vi "Bayer12bit.vi"() -> ()   [LabVIEW 2022 SP3]
uses:
  <vilib>/vision/NI_Vision_Development_Module.lvlib
panel:
  out "Binary Threshold":T1(plugin-control)
  in  "Range":cluster{"Lower value":sgl, "Upper value":sgl}={"Lower value"=128.0, "Upper value"=255.0} {"Upper value" format="%.2f"; "Lower value" format="%.2f"}
  in  "Color Plane":i32(ring)=1 items=["Red", "Green", "Blue", "Hue", "Saturation", "Luminance", "Value", "Intensity"]
  out "Color Plane Extract":T1(plugin-control)
  in  "Bit Depth (0)":u32=12
  out "Processing Time":u32
  in  "RUN":bool
  out "RGB":T1(plugin-control)
  in  "Bayer Parameters":T2={"Pattern"=3, "Algorithm"=0, "Red Gain"=1.0, "Green Gain"=1.0, "Blue Gain"=1.0} {"Blue Gain" format="%_4g"; "Green Gain" format="%_4g"; "Red Gain" format="%_4g"; "Algorithm" items=["Bilinear", "VNG"]; "Pattern" items=["GB", "GR", "BG", "RG"]}
  in  "Stop":bool
  out "Original":T1(plugin-control)
  in  "File Path":path=path "C:/Users/au540322/Documents/Projects/BioDiscover/src/LabVIEW/resources/BayerImages/OriginalBayer.png"
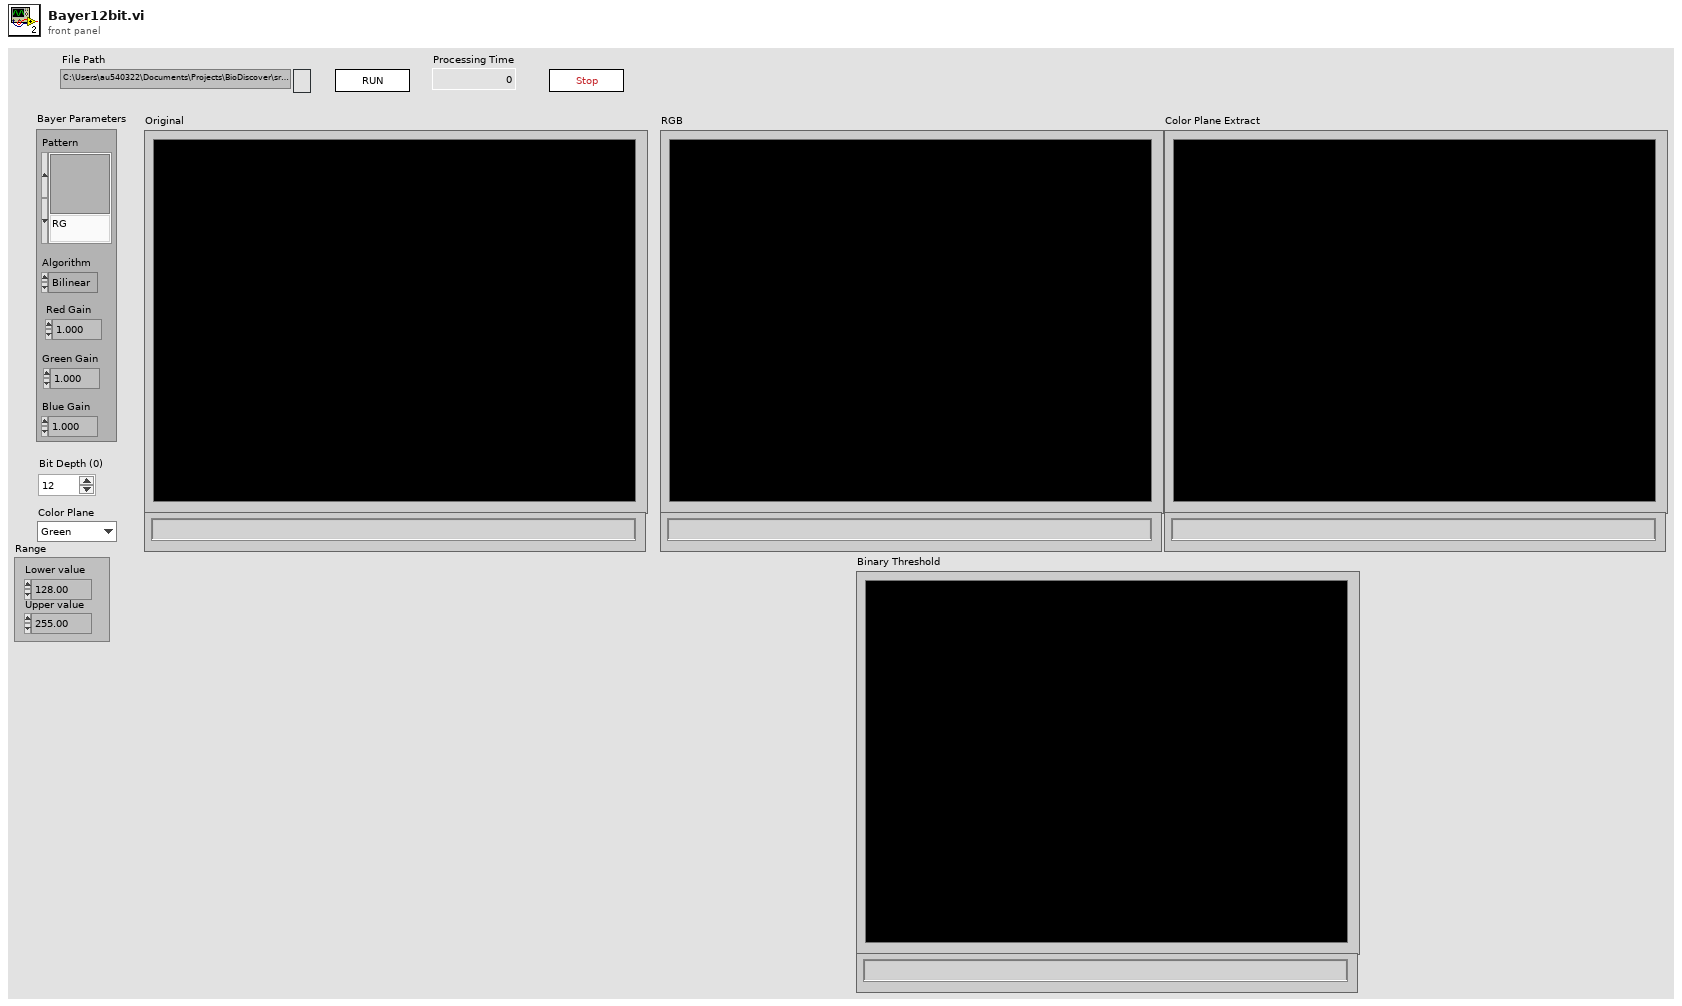
[diagram p1: front panel]
types:
  T1 = typedef "IMAQ Image.ctl" = refnum<image>
  T2 = cluster{"Pattern":i32, "Algorithm":i32, "Red Gain":dbl, "Green Gain":dbl, "Blue Gain":dbl}
  T3 = typedef "Image Type" = u32
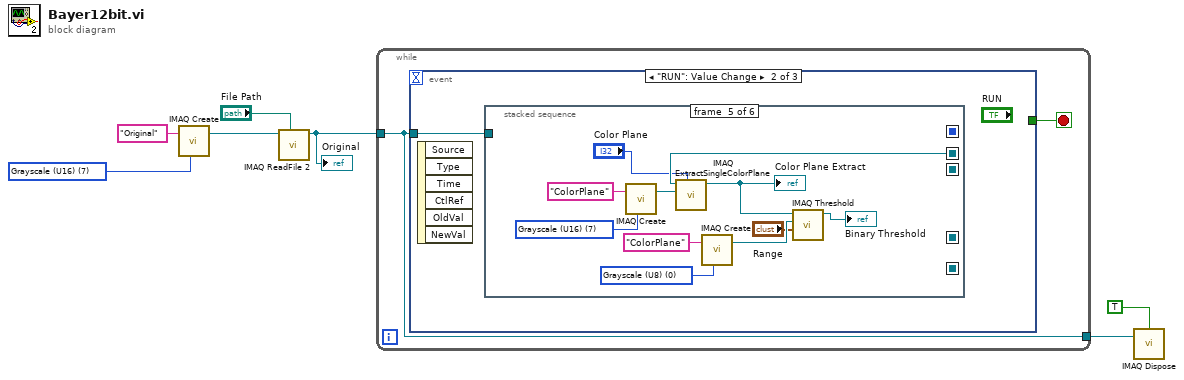
[diagram p0: block diagram]
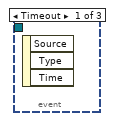
[diagram p2: hidden frame]
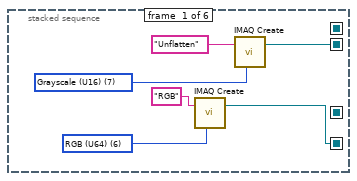
[diagram p3: hidden frame]
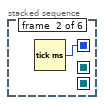
[diagram p4: hidden frame]
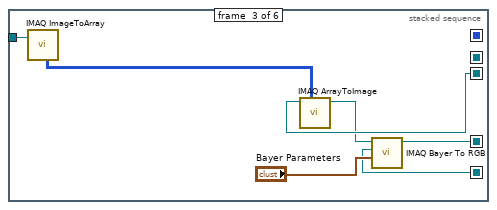
[diagram p5: hidden frame]
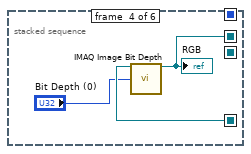
[diagram p6: hidden frame]
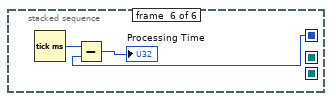
[diagram p7: hidden frame]
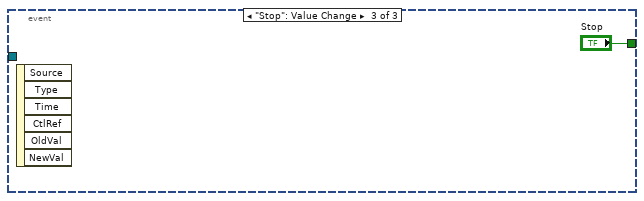
[diagram p8: hidden frame]
diagram:
  w2 = T3 7 items=["Grayscale (U8)", "Grayscale (I16)", "Grayscale (SGL)", "Complex (CSG)", "RGB (U32)", "HSL (U32)", "RGB (U64)", "Grayscale (U16)"] ("Image Type")
  n1 = call "IMAQ Create"("Image Name"="Original", "Image Type"=w2) -> ("New Image"=w6:T1)  [unwired: 3 in, 1 out]
  n2 = call "IMAQ ReadFile 2"("File Path"="File Path", "Image"=w6) -> ("Image Out"=w3:T1)  [unwired: 5 in, 4 out]
  "Original" <- w3
  n3 = while {
    tunnel: w3 -> [w9]
    tunnel: [w9] -> w5
    stop <- w8 stop-if-true
    n4 = event shown="[1] \"RUN\": Value Change" {
      selector: _ -> [_ _ _]
      dyn-events: _ -> [_ _ _]
      timeout: _ -> [_ _ _]
      tunnel: w9 -> [_ w10 _]
      tunnel: [_ _ "Stop"] -> w8
      event Timeout {
        n5 = event-data() -> ()  [unwired: 1 in, 3 out]
      }
      event "RUN": Value Change {
        n6 = event-data() -> ()  [unwired: 1 in, 6 out]
        n7 = stacked-sequence {
          seq-local: [_ w17 _ _ _ _] -> [_ _ _ _ _ w39]
          seq-local: [_ _ w23 _ _ _] -> [_ _ _ w27 _ _]
          seq-local: [_ _ _ w25 _ _] -> [_ _ _ _ w35 _]
          seq-local: [w14 _ _ _ _ _] -> [_ _ w21 _ _ _]
          seq-local: [w11 _ _ _ _ _] -> [_ _ w18 _ _ _]
          tunnel: w10 -> [_ _ w22 _ _ _]
          frame #0 {
            w13 = T3 6 items=["Grayscale (U8)", "Grayscale (I16)", "Grayscale (SGL)", "Complex (CSG)", "RGB (U32)", "HSL (U32)", "RGB (U64)", "Grayscale (U16)"] ("Image Type")
            w15 = T3 7 items=["Grayscale (U8)", "Grayscale (I16)", "Grayscale (SGL)", "Complex (CSG)", "RGB (U32)", "HSL (U32)", "RGB (U64)", "Grayscale (U16)"] ("Image Type")
            n8 = call "IMAQ Create"("Image Name"="RGB", "Image Type"=w13) -> ("New Image"=w11:T1)  [unwired: 3 in, 1 out]
            n9 = call "IMAQ Create"("Image Name"="Unflatten", "Image Type"=w15) -> ("New Image"=w14:T1)  [unwired: 3 in, 1 out]
          }
          frame #1 {
            n10 = Tick Count (ms)() -> (millisecond timer value=w17:u32)
          }
          frame #2 {
            n11 = call "IMAQ ImageToArray"("Image"=w22) -> ("Image Pixels (U16)"=w19:u16[][])  [unwired: 3 in, 4 out]
            n12 = call "IMAQ ArrayToImage"("Image Pixels (U16)"=w19, "Image"=w21) -> ("Image Out"=w20:T1)  [unwired: 8 in, 1 out]
            n13 = call "IMAQ Bayer To RGB"("Bayer Parameters"="Bayer Parameters", "Image Dst"=w18, "Image Src"=w20) -> ("Image Dst Out"=w23:T1)  [unwired: 7 in, 1 out]
          }
          frame #3 {
            n14 = call "IMAQ Image Bit Depth"("Image"=w27, "Bit Depth (0)"="Bit Depth (0)") -> ("Image Out"=w25:T1)  [unwired: 11 in, 2 out]
            "RGB" <- w25
          }
          frame #4 {
            w28 = T3 0 items=["Grayscale (U8)", "Grayscale (I16)", "Grayscale (SGL)", "Complex (CSG)", "RGB (U32)", "HSL (U32)", "RGB (U64)", "Grayscale (U16)"] ("Image Type")
            w37 = T3 7 items=["Grayscale (U8)", "Grayscale (I16)", "Grayscale (SGL)", "Complex (CSG)", "RGB (U32)", "HSL (U32)", "RGB (U64)", "Grayscale (U16)"] ("Image Type")
            n15 = call "IMAQ Create"("Image Name"="ColorPlane", "Image Type"=w37) -> ("New Image"=w36:T1)  [unwired: 3 in, 1 out]
            n16 = call "IMAQ ExtractSingleColorPlane"("Color Plane"="Color Plane", "Image Dst"=w36, "Image Src"=w35) -> ("Image Dst Out"=w33:T1)  [unwired: 1 in, 7 out]
            "Color Plane Extract" <- w33
            n17 = call "IMAQ Create"("Image Name"="ColorPlane", "Image Type"=w28) -> ("New Image"=w31:T1)  [unwired: 3 in, 1 out]
            n18 = call "IMAQ Threshold"("Range"="Range", "Image Dst"=w31, "Image Src"=w33) -> ("Image Dst Out"=→"Binary Threshold":T1)  [unwired: 7 in, 1 out]
          }
          frame #5 {
            n19 = Tick Count (ms)() -> (millisecond timer value=w41:u32)
            n20 = Subtract(x=w41, y=w39) -> (x-y=→"Processing Time":u32)
          }
        }
      }
      event "Stop": Value Change {
        n21 = event-data() -> ()  [unwired: 1 in, 6 out]
      }
    }
  }
  n22 = call "IMAQ Dispose"("All Images? (No)"=TRUE, "Image"=w5) -> ()  [unwired: 4 in, 1 out]
